vi "DVR Creator.vi"(0 "Numeric (double)":dbl, 5 "Increment":bool, 11 "error in":errorcluster) -> (15 "error out":errorcluster)   [LabVIEW 2023]
doc: "DVR creatr VI gets the numeric double input from the user and when increment button is pressed, DVR reference is stored in the LV2 and when New DVR VI is runned and pressed the corresponding booelan, numeric value incremented in the current VI is displayed in the New DVR VI only when the current VI is in running state."
uses:
  LV2/Controls/LV2Operations.ctl
panel:
  in  "Stop":bool
  # "INSTRUCTIONS:\n\n1. Run the VI.\n2. Enter value in Numeric(double) control.\n3. Press INCREMENT button to increment the \n    numeric input.\n4. Run New DVR VI and press Read DVR Value \n    to display the value incremented from the current VI.\n5. Press Stop or close the Front Panel to abort the VI."
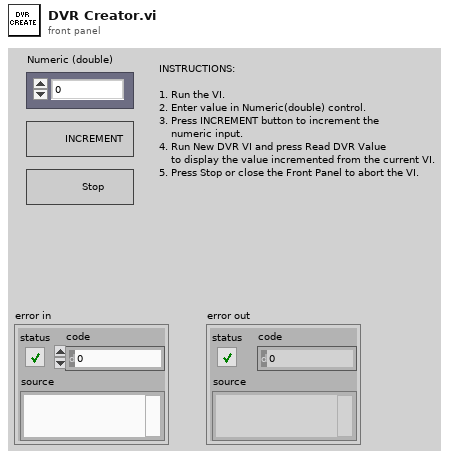
[diagram p1: front panel]
types:
  T1 = enum8{"Enabled", "Disabled", "Disabled and Grayed Out"}
  T2 = typedef "LV2Operations.ctl" = enum16{"Init", "Read", "Write"}
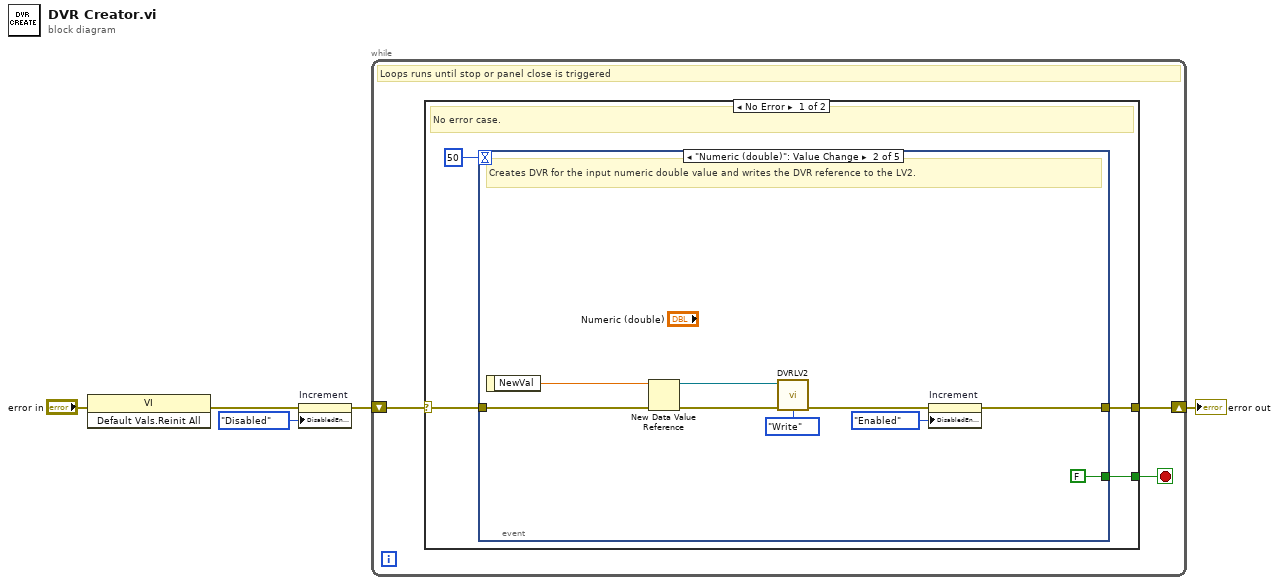
[diagram p0: block diagram]
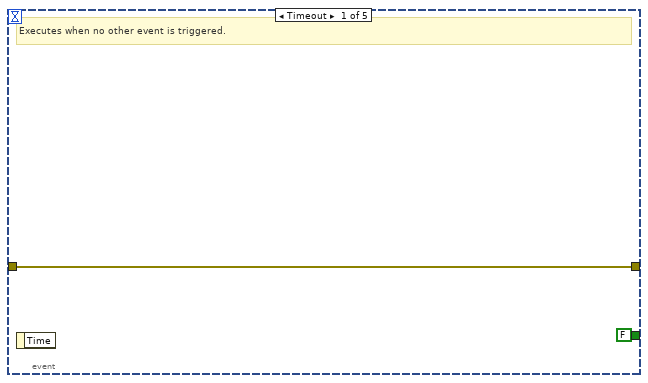
[diagram p2: hidden frame]
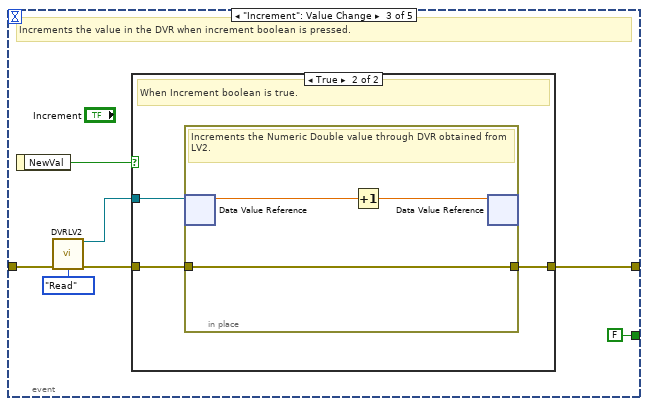
[diagram p3: hidden frame]
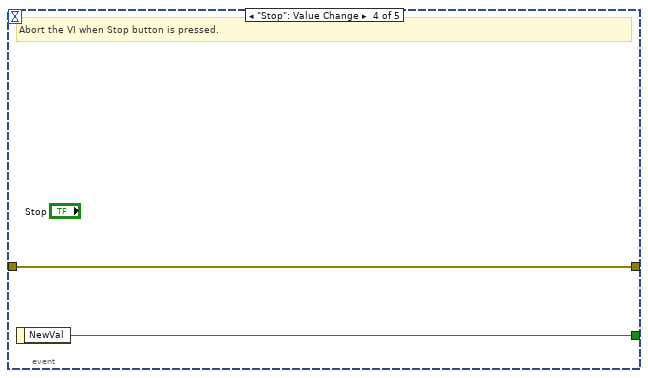
[diagram p5: hidden frame]
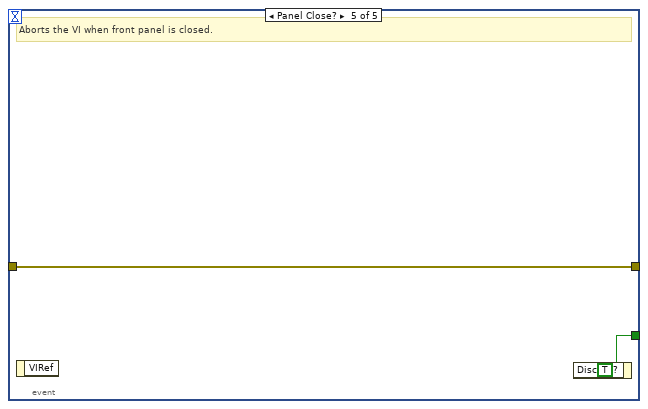
[diagram p6: hidden frame]
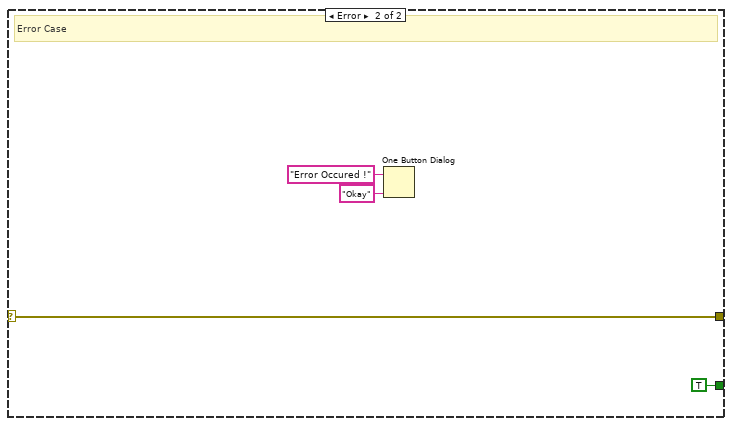
[diagram p7: hidden frame]
diagram:
  n1 = invoke class="VI" method="Default Vals.Reinit All"(error in="error in") -> (error out=w2:errorcluster)  [unwired: 2 in, 2 out]
  n2 = property on="Increment" class="Bool"(error in=w2, "DisabledEnum"=T1."Disabled" ("Disabled")) -> (error out=w1:errorcluster)  [unwired: 1 in, 1 out]
  n3 = while {
    shift-right: [w7] -> w4
    shift-left: w1 -> [w8]
    stop <- w6 stop-if-true
    # "Loops runs until stop or panel close is triggered"
    n4 = case shown="No Error" w8 {
      selector: w8 -> [w11 w45]
      tunnel: [w10 w45] -> w7
      tunnel: [w9 TRUE ("Discard?")] -> w6
      frame No Error {
        # "No error case."
        n5 = event shown="[1] \"Numeric (double)\": Value Change" {
          selector: _ -> [_ _ _ _ _]
          dyn-events: _ -> [_ _ _ _ _]
          timeout: 50 -> [_ _ _ _ _]
          tunnel: w11 -> [w13 w22 w26 w38 w40]
          tunnel: [w13 w16 w29 w38 w40] -> w10
          tunnel: [FALSE FALSE FALSE w39 w41] -> w9
          event Timeout {
            # "Executes when no other event is triggered."
            n6 = event-data() -> ()  [unwired: 1 in, 1 out]
          }
          event "Numeric (double)": Value Change {
            # "Creates DVR for the input numeric double value and writes the DVR reference to the LV2."
            n7 = event-data() -> ("NewVal"=w23:dbl)  [unwired: 1 in]
            n8 = New Data Value Reference(data value=w23, error in=w22) -> (data value reference=w17:refnum<data-value>, error out=w20:errorcluster)
            n9 = call "DVRLV2.vi"("data value reference in"=w17, "error in"=w20, "Operations"=LV2Operations."Write") -> ("error out"=w19:errorcluster)  [unwired: 11 in, 1 out]
            n10 = property on="Increment" class="Bool"(error in=w19, "DisabledEnum"=T1."Enabled" ("Disabled")) -> (error out=w16:errorcluster)  [unwired: 1 in, 1 out]
          }
          event "Increment": Value Change {
            # "Increments the value in the DVR when increment boolean is pressed."
            n11 = event-data() -> ("NewVal"=w30:bool)  [unwired: 1 in]
            n12 = call "DVRLV2.vi"("error in"=w26, "Operations"=LV2Operations."Read") -> ("data value reference out"=w24:refnum<data-value>, "error out"=w25:errorcluster)  [unwired: 12 in]
            n13 = case shown="True" w30 {
              tunnel: w25 -> [w31 w34]
              tunnel: [w31 w33] -> w29
              tunnel: w24 -> [_ w32]
              frame False {
                # "When Increment boolean is false."
              }
              frame True {
                # "When Increment boolean is true."
                n14 = in-place {
                  in-place-border: w34 -> [w37]
                  in-place-border: [w37] -> w33
                  # "Increments the Numeric Double value through DVR obtained from LV2."
                  n15 = in-place-dvr #1(w32) -> (w36:dbl)  [unwired: 1 out]
                  n16 = Increment(x=w36) -> (x+1=w35:dbl)
                  n17 = in-place-dvr #1(w35) -> ()  [unwired: 2 out]
                }
              }
            }
          }
          event "Stop": Value Change {
            # "Abort the VI when Stop button is pressed."
            n18 = event-data() -> ("NewVal"=w39:bool)  [unwired: 1 in]
          }
          event Panel Close? {
            w41 = TRUE ("Discard?")
            # "Aborts the VI when front panel is closed."
            n19 = event-data() -> ()  [unwired: 1 in, 1 out]
            n20 = event-data("Discard?"=w41) -> ()  [unwired: 1 in, 1 out]
          }
        }
      }
      frame Error {
        # "Error Case"
        n21 = One Button Dialog(message="Error Occured !", button name ("OK")="Okay") -> ()  [unwired: 1 out]
      }
    }
  }
  "error out" <- w4
